vi "Set Special.vi"(8 "error in (no error)":errorcluster, 10 "Special":bool, 11 "FrameworkSubTestSuite in":refnum<class "FrameworkSubTestSuite.lvclass">) -> (0 "error out":errorcluster, 3 "FrameworkSubTestSuite out":refnum<class "FrameworkSubTestSuite.lvclass">)   [LabVIEW 2013, in "FrameworkSubTestSuite.lvclass"]
uses:
  FrameworkSubTestSuite.lvclass
  FrameworkSubTestSuite.lvclass/FrameworkSubTestSuite.ctl
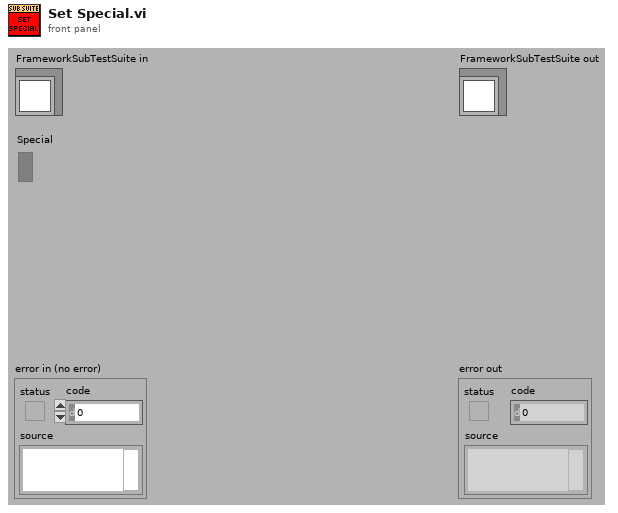
[diagram p1: front panel]
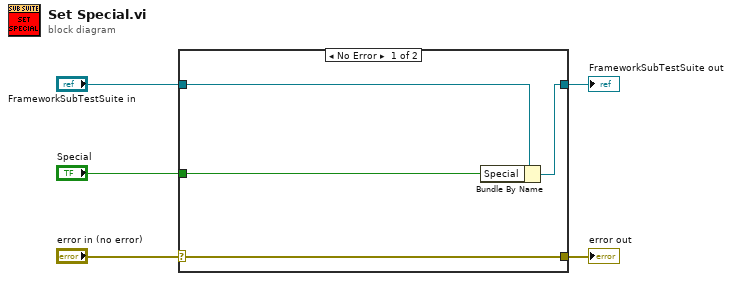
[diagram p0: block diagram]
diagram:
  n1 = case shown="No Error" "error in (no error)" {
    selector: "error in (no error)" -> [w9 w10]
    tunnel: [w9 w10] -> w4
    tunnel: [w7 w11] -> w2
    tunnel: "FrameworkSubTestSuite in" -> [w8 w11]
    tunnel: "Special" -> [w6 _]
    frame No Error {
      n2 = Bundle By Name(cluster=w8, "Special"=w6) -> (w7:refnum<class "FrameworkSubTestSuite.lvclass">)
    }
    frame Error {
    }
  }
  "error out" <- w4
  "FrameworkSubTestSuite out" <- w2
